vi "Photo Current of solar cell (SubVI).vi"(6 "G":dbl, 9 "I_sc":dbl, 10 "k_i":dbl, 11 "T":dbl) -> (3 "I_ph":dbl)   [LabVIEW 2024]
panel:
  # "I ph = [ I sc + k i .( T − 298)].G/1000"
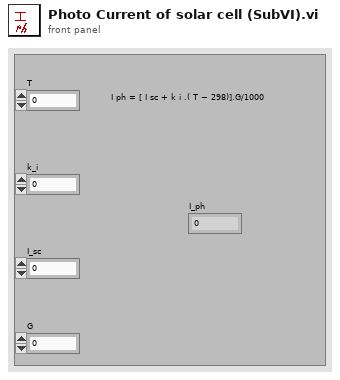
[diagram p1: front panel]
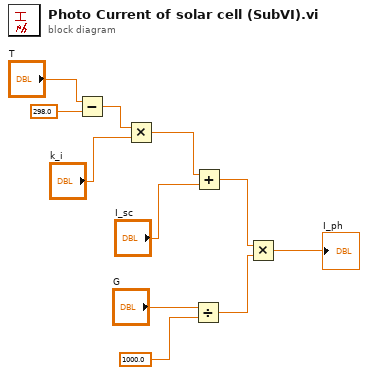
[diagram p0: block diagram]
diagram:
  n1 = Subtract(x="T", y=298.0) -> (x-y=w5:dbl)
  n2 = Multiply(x=w5, y="k_i") -> (x*y=w7:dbl)
  n3 = Divide(x="G", y=1000.0) -> (x/y=w10:dbl)
  n4 = Add(x=w7, y="I_sc") -> (x+y=w9:dbl)
  n5 = Multiply(x=w9, y=w10) -> (x*y=→"I_ph":dbl)
